vi "GUI Manager Module.vi"(8 "Error In":errorcluster) -> (0 "Error Out":errorcluster)   [LabVIEW 2022 SP3]
doc: "This is the GUI Manager Module. It is an asynchronous module that takes commands via a queue.\n\nIt is responsible for initialising the following tickboxes, and maintaining them in a consistent state:\nAdd to Project?\nAdd to Owner?\nAdd to Virtual Folder?\n\nA module is necessary because initialising and maintaining the tickboxes is a relatively complex task."
uses:
  Module Data.ctl
  GUI Object Refs (cluster).ctl
  Input Conditions (cluster).ctl
  Initial State (enum).ctl
  DFS Output (cluster).ctl
panel:
  out "MHL iteration":i32
  # "This is an asynchronous, queue-driven module.\nThis module uses a single loop:\na Message Handling Loop (queue driven)"
  # "Input\nInputs to the VI"
  # "Development\ncontrols/indicators useful for development and testing, but which are not outputs of the VI"
  # "Output\nOutputs of the VI"
  # "The Error Out indicator is larger than usual in order to be able to view the full error message without having to scroll."
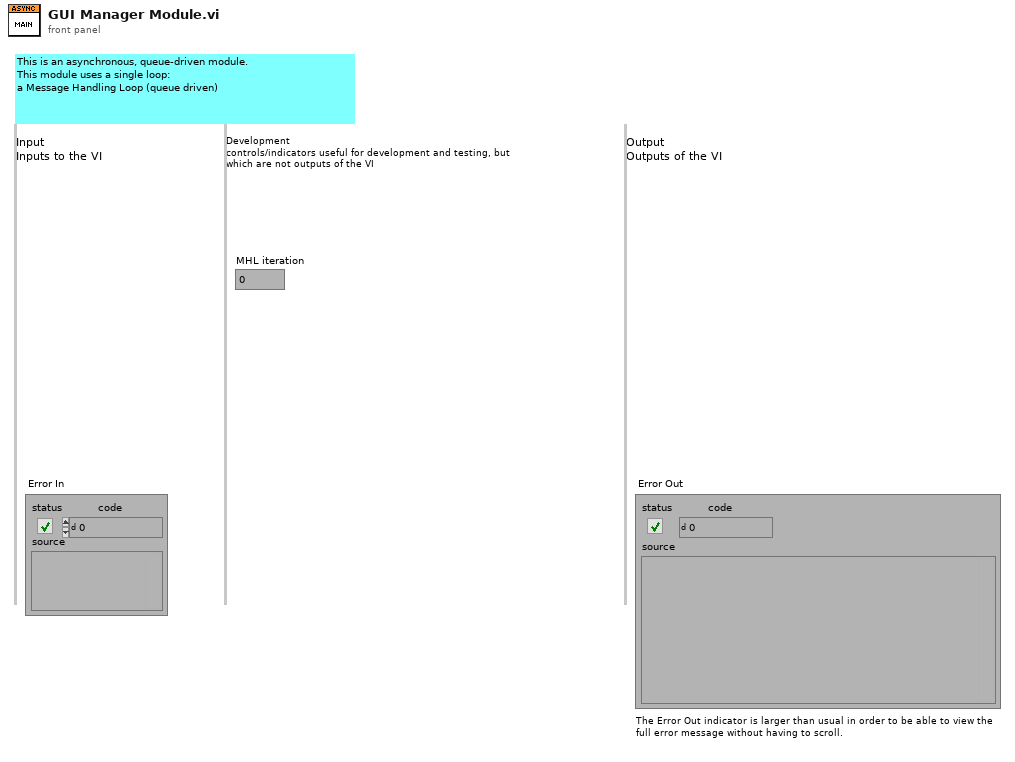
[diagram p1: front panel]
types:
  T1 = typedef "Module Data.ctl" = cluster{"GUI Objects":T2, "Input Conditions":T3, "Initial State":T5}
  T2 = typedef "GUI Object Refs (cluster).ctl" = cluster{"SCL":refnum<vi>, "Add To Owner?":refnum<vi>, "Add To Project?":refnum<vi>, "Open Front Panel?":refnum<vi>, "Destination Folder":refnum<vi>, "Create Button":refnum<vi>, "Project Name ComboBox":refnum<vi>, "NoTemplatesFound Message":refnum<vi>, "Diagram Preview Subpanel":refnum<vi>, "Add to Virtual Folder?":refnum<vi>, "Virtual Folder Path":refnum<vi>, "New Filename":refnum<vi>, "VI Description":refnum<vi>, "Initial State Indicator":refnum<vi>}
  T3 = typedef "Input Conditions (cluster).ctl" = cluster{"Exactly one lvproj open?":bool, "Multiple lvproj open?":bool, "Is User VI owned?":bool, "Is User VI inside virtual folder?":bool, "Owner Filename":string, "Virtual Folder Search Results":T4, "Project Names":string[]}
  T4 = typedef "DFS Output (cluster).ctl" = cluster{"Was VI Found?":bool, "Was VI Found Inside Virtual Folder?":bool, "Project Item Ref (The VI)":refnum<vi>, "Project Item Ref (Containing Folder)":refnum<vi>, "Folder Path":string, "Was Search Aborted?":bool}
  T5 = typedef "Initial State (enum).ctl" = enum16{"Initial State 0", "Initial State 1", "Initial State 2", "Initial State 3", "Initial State 4", "Initial State 5", "Initial State 6", "Initial State 7", "Initial State 8", "Initial State 9", "Initial State 10", "Initial State 11", "Initial State 12", "Initial State 13", "Initial State 14", "Initial State 15"}
  T6 = typedef "Command.ctl" = enum16{"Init Module", "Shutdown Module", "Local Error Handler", "Init Tickboxes", "Handle Value Change - Add to Project", "Handle Value Change - Add to Owner", "Handle Value Change - Add to Virtual Folder"}
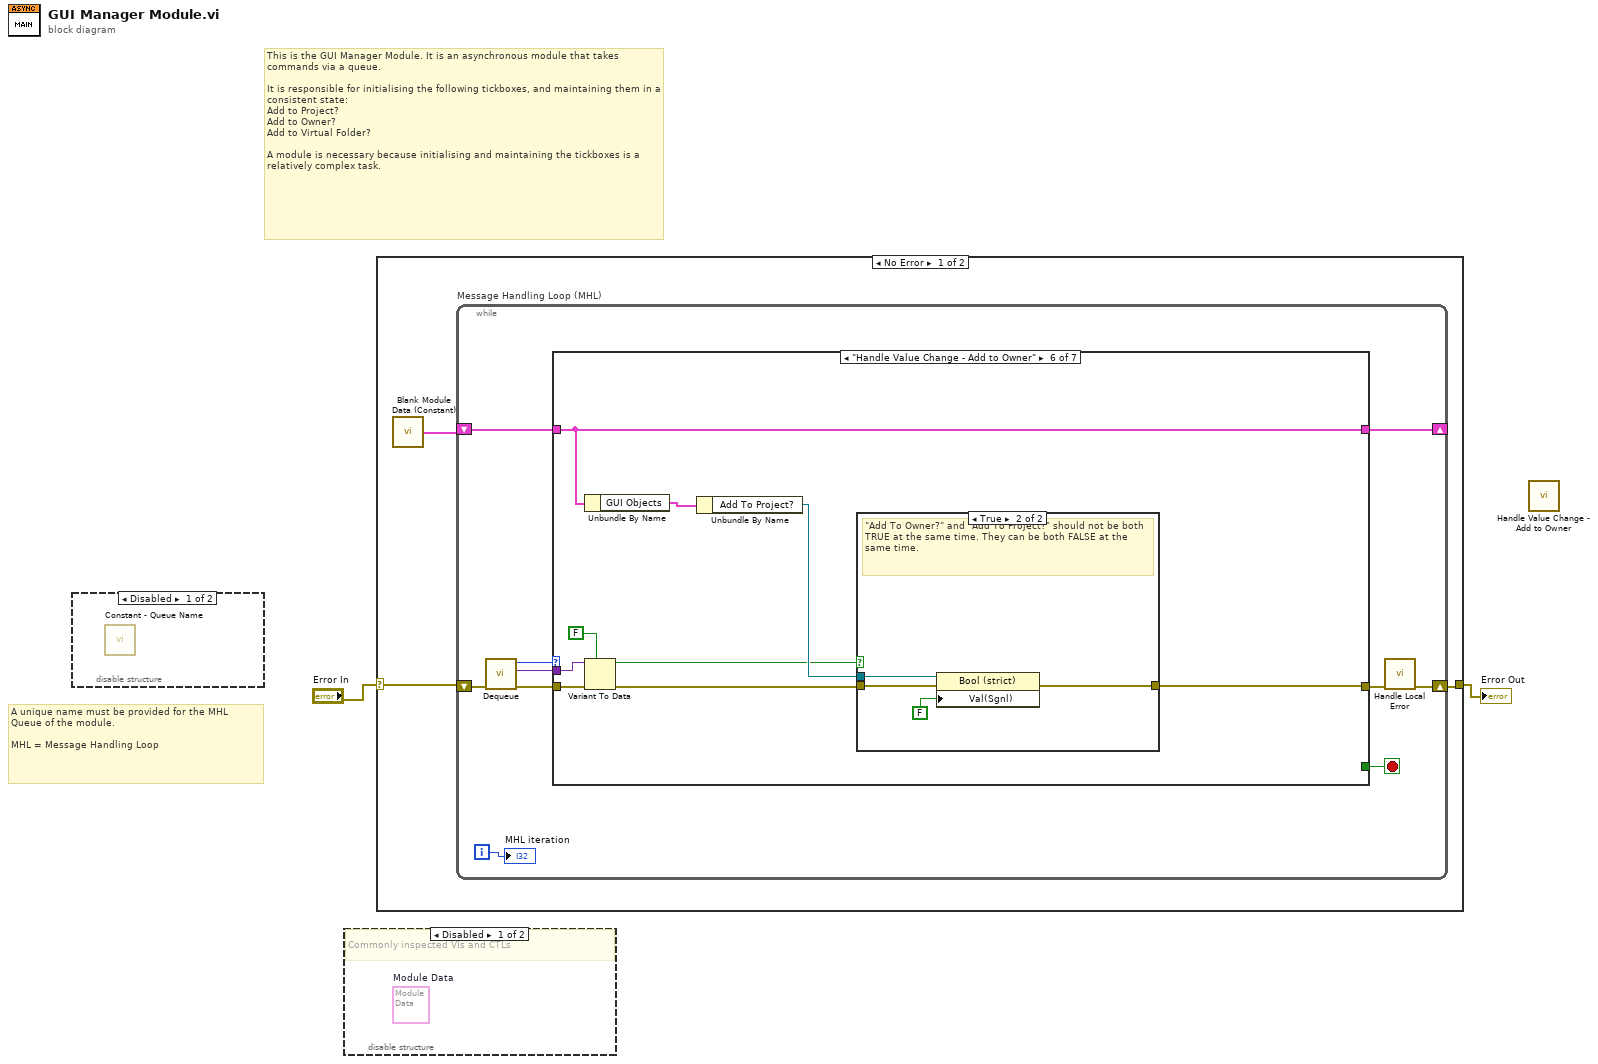
[diagram p0: block diagram]
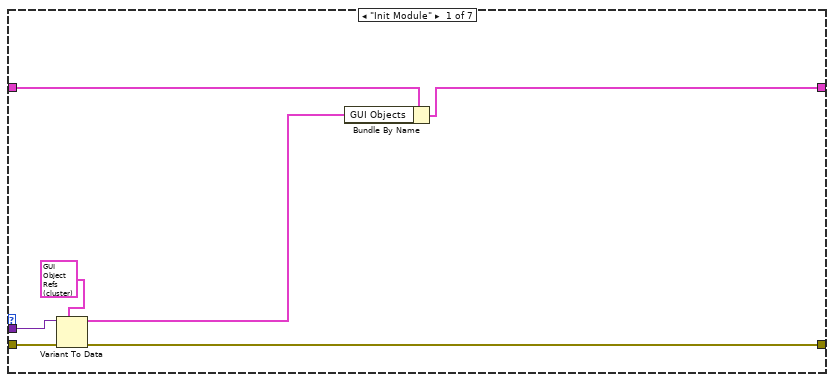
[diagram p2: hidden frame]
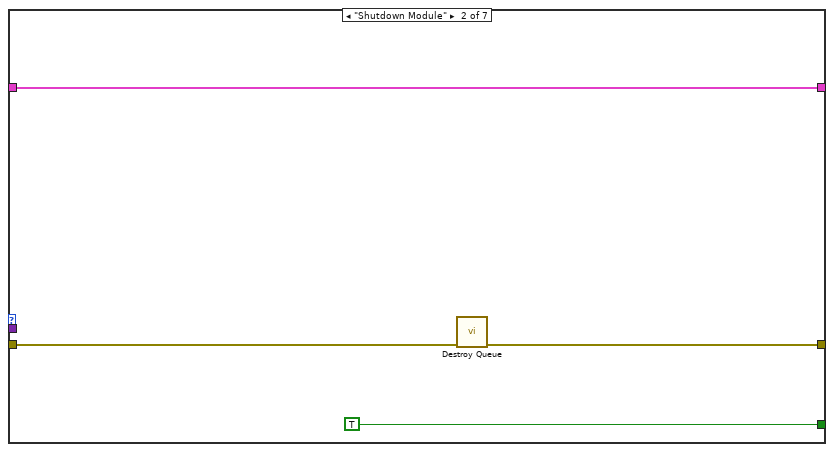
[diagram p3: hidden frame]
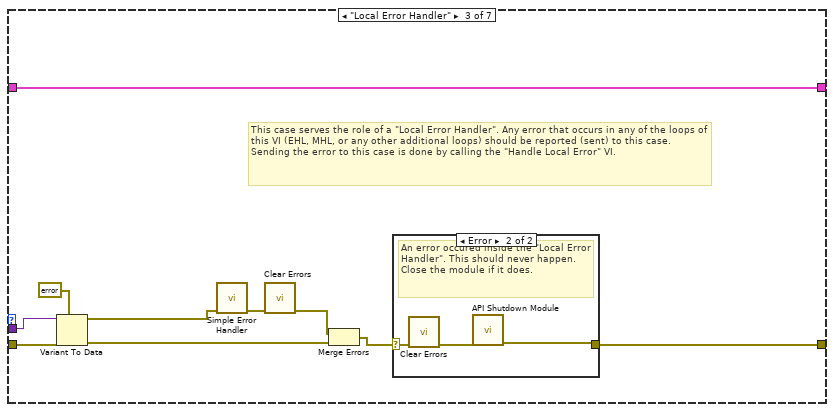
[diagram p4: hidden frame]
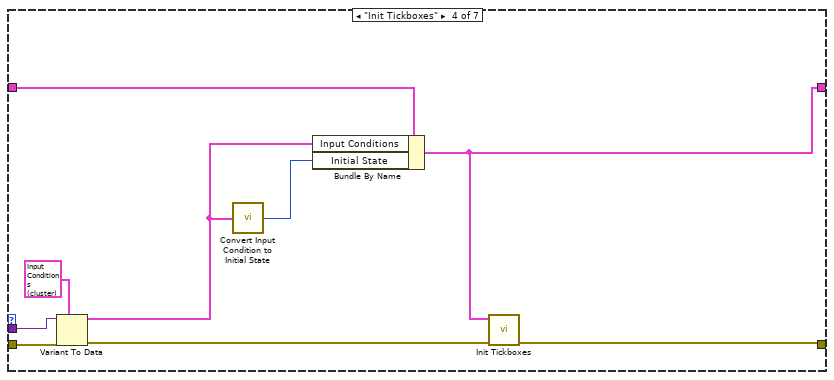
[diagram p6: hidden frame]
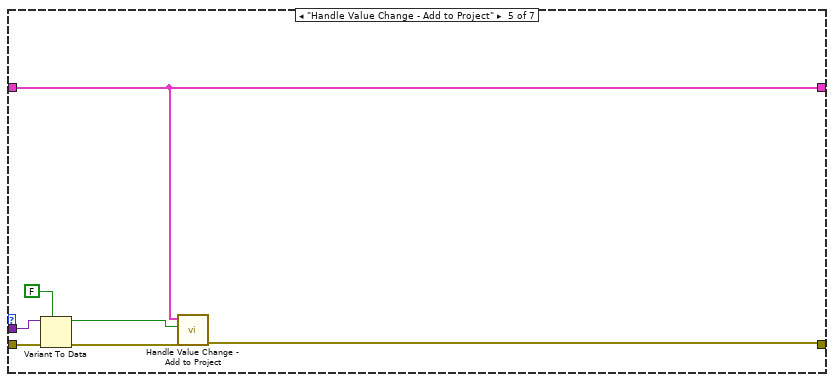
[diagram p7: hidden frame]
diagram:
  # "A unique name must be provided for the MHL Queue of the module.\n\nMHL = Message Handling Loop"
  # "This is the GUI Manager Module. It is an asynchronous module that takes commands via a queue.\n\nIt is responsible for initialising the following tickboxes, and maintaining them in a consistent state:\nAdd to Project?\nAdd to Owner?\nAdd to Virtual Folder?\n\nA module is necessary because initialising and maintaining the tickboxes is a relatively complex task."
  n1 = disable-structure shown="Disabled" {
    frame Disabled {
      n2 = call "Constant - Queue Name.vi"() -> ()  [unwired: 1 out]
    }
    frame Enabled {
    }
  }
  n3 = disable-structure shown="Disabled" {
    frame Disabled {
      (unwired) T1 {"GUI Objects"={"SCL"=refnum, "Add To Owner?"=refnum, "Add To Project?"=refnum, "Open Front Panel?"=refnum, "Destination Folder"=refnum, "Create Button"=refnum, "Project Name ComboBox"=refnum, "NoTemplatesFound Message"=refnum, "Diagram Preview Subpanel"=refnum, "Add to Virtual Folder?"=refnum, "Virtual Folder Path"=refnum, "New Filename"=refnum, "VI Description"=refnum, "Initial State Indicator"=refnum}, "Input Conditions"={"Exactly one lvproj open?"=FALSE, "Multiple lvproj open?"=FALSE, "Is User VI owned?"=FALSE, "Is User VI inside virtual folder?"=FALSE, "Owner Filename"="", "Virtual Folder Search Results"={"Was VI Found?"=FALSE, "Was VI Found Inside Virtual Folder?"=FALSE, "Project Item Ref (The VI)"=refnum, "Project Item Ref (Containing Folder)"=refnum, "Folder Path"="", "Was Search Aborted?"=FALSE}, "Project Names"=[]}, "Initial State"=enum."Initial State 0"}  # Module Data
      # "Commonly inspected VIs and CTLs"
    }
    frame Enabled {
    }
  }
  n4 = case shown="No Error" "Error In" {
    selector: "Error In" -> [w3 w73]
    tunnel: [w5 w73] -> w2
    frame No Error {
      n5 = call "Blank Module Data (Constant).vi"() -> ("Blank Module Data"=w4:T1)
      n6 = while "Message Handling Loop (MHL)" {
        shift-right: [w8] -> _
        shift-left: w4 -> [w7]
        shift-right: [w12] -> w5
        shift-left: w3 -> [w11]
        i -> [w9]
        stop <- w15 stop-if-true
        n7 = call "Dequeue.vi"("error in (no error)"=w11) -> ("error out"=w13:errorcluster, "Data"=w10:variant, "Command"=w6:T6)  [unwired: 8 in]
        n8 = case shown="\"Handle Value Change - Add to Owner\"" w6 {
          tunnel: w13 -> [w20 w26 w30 w49 w56 w65 w72]
          tunnel: [w19 w25 w28 w42 w50 w59 w72] -> w14
          tunnel: [_ TRUE _ _ _ _ _] -> w15
          tunnel: w10 -> [w18 _ w29 w48 w55 w62 _]
          tunnel: [w21 w24 w36 w41 w51 w64 w71] -> w8
          tunnel: w7 -> [w22 w24 w36 w46 w51 w64 w71]
          frame "Init Module" {
            n9 = Variant To Data(error in=w20, type=T2 {"SCL"=refnum, "Add To Owner?"=refnum, "Add To Project?"=refnum, "Open Front Panel?"=refnum, "Destination Folder"=refnum, "Create Button"=refnum, "Project Name ComboBox"=refnum, "NoTemplatesFound Message"=refnum, "Diagram Preview Subpanel"=refnum, "Add to Virtual Folder?"=refnum, "Virtual Folder Path"=refnum, "New Filename"=refnum, "VI Description"=refnum, "Initial State Indicator"=refnum} ("GUI Objects"), Variant=w18) -> (data=w16:T2, error out=w19:errorcluster)
            n10 = Bundle By Name(cluster=w22, "GUI Objects"=w16) -> (w21:T1)
          }
          frame "Shutdown Module" {
            n11 = call "Destroy Queue.vi"("error in (no error)"=w26) -> ("error out"=w25:errorcluster)  [unwired: 8 in, 2 out]
          }
          frame "Local Error Handler" {
            # "This case serves the role of a \"Local Error Handler\". Any error that occurs in any of the loops of this VI (EHL, MHL, or any other additional loops) should be reported (sent) to this case. Sending the error to this case is done by calling the \"Handle Local Error\" VI."
            n12 = Variant To Data(error in=w30, type=errorcluster {"status"=FALSE, "code"=0, "source"=""} ("error constant"), Variant=w29) -> (data=w33:errorcluster, error out=w32:errorcluster)
            n13 = call <vilib>:"Simple Error Handler.vi"("error in (no error)"=w33) -> ("error out"=w34:errorcluster)  [unwired: 4 in, 4 out]
            n14 = call <vilib>:"Clear Errors.vi"("error in (no error)"=w34) -> ("error out"=w27:errorcluster)  [unwired: 5 in, 1 out]
            n15 = Merge Errors(w27, w32) -> (w31:errorcluster)
            n16 = case shown="Error" w31 {
              selector: w31 -> [w37 w40]
              tunnel: [w37 w39] -> w28
              frame No Error {
                # "Desired. Expected to always execute."
              }
              frame Error {
                # "An error occured inside the \"Local Error Handler\". This should never happen. Close the module if it does."
                n17 = call <vilib>:"Clear Errors.vi"("error in (no error)"=w40) -> ("error out"=w38:errorcluster)  [unwired: 5 in, 1 out]
                n18 = call "API Shutdown Module.vi"("Error In"=w38) -> ("Error Out"=w39:errorcluster)  [unwired: 10 in]
              }
            }
          }
          frame "Init Tickboxes" {
            n19 = Variant To Data(error in=w49, type=T3 {"Exactly one lvproj open?"=FALSE, "Multiple lvproj open?"=FALSE, "Is User VI owned?"=FALSE, "Is User VI inside virtual folder?"=FALSE, "Owner Filename"="", "Virtual Folder Search Results"={"Was VI Found?"=FALSE, "Was VI Found Inside Virtual Folder?"=FALSE, "Project Item Ref (The VI)"=refnum, "Project Item Ref (Containing Folder)"=refnum, "Folder Path"="", "Was Search Aborted?"=FALSE}, "Project Names"=[]} ("Input Conditions"), Variant=w48) -> (data=w45:T3, error out=w43:errorcluster)
            n20 = call "Convert Input Condition to Initial State.vi"("Input Conditions"=w45) -> ("Initial State"=w44:T5)
            n21 = Bundle By Name(cluster=w46, "Input Conditions"=w45, "Initial State"=w44) -> (w41:T1)
            n22 = call "Init Tickboxes.vi"("Error In"=w43, "Module Data"=w41) -> ("Error Out"=w42:errorcluster)  [unwired: 9 in]
          }
          frame "Handle Value Change - Add to Project" {
            n23 = Variant To Data(error in=w56, type=FALSE, Variant=w55) -> (data=w52:bool, error out=w53:errorcluster)
            n24 = call "Handle Value Change - Add to Project.vi"("Error In"=w53, "New Value"=w52, "Module Data In"=w51) -> ("Error Out"=w50:errorcluster)  [unwired: 8 in]
          }
          frame "Handle Value Change - Add to Owner" {
            n25 = Unbundle By Name(w64) -> ("GUI Objects"=w63:T2)
            n26 = Variant To Data(error in=w65, type=FALSE, Variant=w62) -> (data=w57:bool, error out=w60:errorcluster)
            n27 = Unbundle By Name(w63) -> ("Add To Project?"=w58:refnum<vi>)
            n28 = case shown="True" w57 {
              tunnel: w60 -> [w66 w70]
              tunnel: [w66 w69] -> w59
              tunnel: w58 -> [_ w67]
              frame False {
              }
              frame True {
                # "\"Add To Owner?\" and \"Add To Project?\" should not be both TRUE at the same time. They can be both FALSE at the same time."
                n29 = property class="Bool (strict)"(reference=w67, error in=w70, "Val(Sgnl)"=FALSE ("Value (Signaling)")) -> (error out=w69:errorcluster)  [unwired: 1 out]
              }
            }
          }
          frame "Handle Value Change - Add to Virtual Folder" {
          }
        }
        n30 = call "Handle Local Error.vi"("Error In"=w14) -> ("Error Out"=w12:errorcluster)  [unwired: 10 in]
        "MHL iteration" <- w9
      }
    }
    frame Error {
    }
  }
  "Error Out" <- w2
  n31 = call "Handle Value Change - Add to Owner.vi"() -> ()  [unwired: 11 in, 1 out]
